vi "cdaq_test.vi"() -> ()   [LabVIEW 2013]
uses:
  cdaq_anal_session.ctl
  cdaq_anal_adc_command.ctl
  cdaq_anal_adc_data.ctl
panel:
  out "error out 2":errorcluster
  out "timestamp [s]":dbl
  out "adc data":dbl[](graph)
  in  "ADC N":i32
  in  "btn adc get":bool
  in  "btn set dac":bool
  in  "amp":sgl
  in  "ws":sgl
  in  "N":i32
  in  "btn stop":bool
  out "error out":errorcluster
  in  "cdaq session in":T1={"mclk [Hz]"=12800000.0, "DAC device"="cDAQ2Mod7", "ADC device"="cDAQ2Mod8", "DAC task"="", "ADC task"="", "adc idn"="", "dac idn"="", "fs [Hz]"=50000.0, "queue adc cmd"=refnum, "queue adc data"=refnum, "adc proc ref"=refnum}
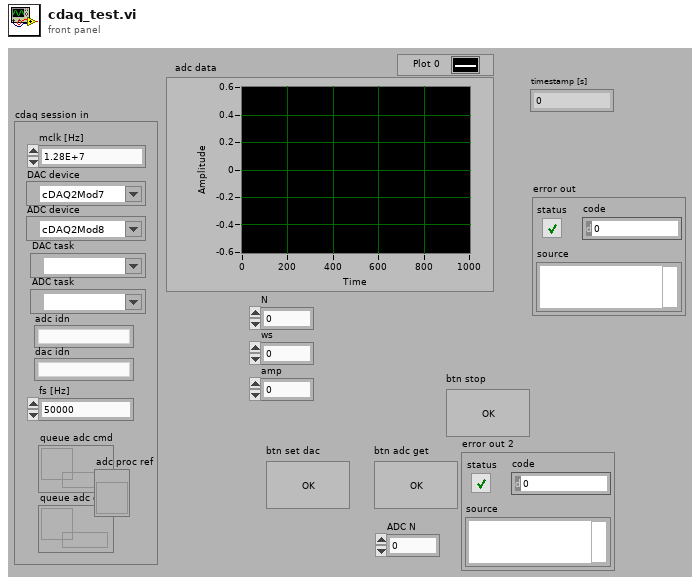
[diagram p1: front panel]
types:
  T1 = typedef "cdaq_anal_session.ctl" = cluster{"mclk [Hz]":dbl, "DAC device":tag, "ADC device":tag, "DAC task":refnum<k21>, "ADC task":refnum<k21>, "adc idn":string, "dac idn":string, "fs [Hz]":dbl, "queue adc cmd":refnum<queue>, "queue adc data":refnum<queue>, "adc proc ref":refnum<vi>}
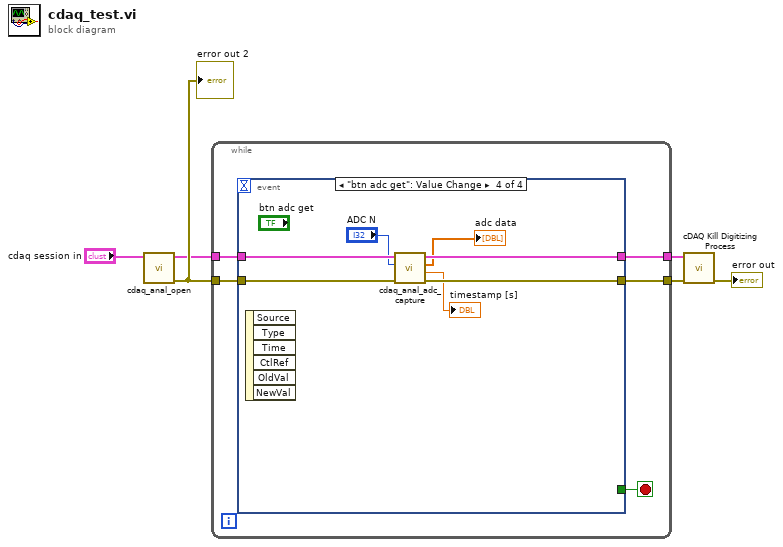
[diagram p0: block diagram]
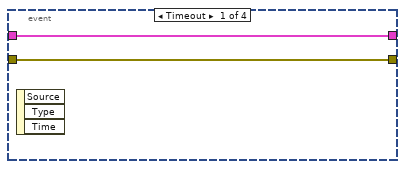
[diagram p2: hidden frame]
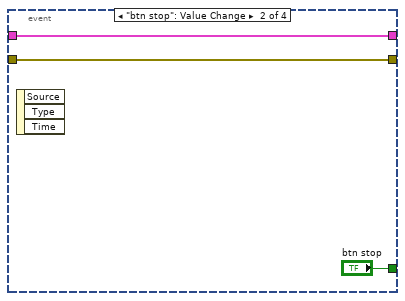
[diagram p3: hidden frame]
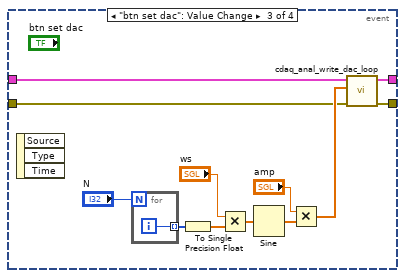
[diagram p4: hidden frame]
diagram:
  n1 = call "cdaq_anal_open.vi"("cdaq session in"="cdaq session in") -> ("error out"=w3:errorcluster, "cdaq session out"=w2:T1)  [unwired: 7 in, 2 out]
  "error out 2" <- w3
  n2 = while {
    tunnel: [w11] -> w5
    tunnel: w3 -> [w10]
    tunnel: w2 -> [w9]
    tunnel: [w8] -> w1
    stop <- w7 stop-if-true
    n3 = event shown="[3] \"btn adc get\": Value Change" {
      selector: _ -> [_ _ _ _]
      dyn-events: _ -> [_ _ _ _]
      timeout: _ -> [_ _ _ _]
      tunnel: [w13 w15 w20 w34] -> w11
      tunnel: w10 -> [w13 w15 w19 w36]
      tunnel: w9 -> [w12 w16 w18 w35]
      tunnel: [w12 w16 w17 w33] -> w8
      tunnel: [_ "btn stop" _ _] -> w7
      event Timeout {
        n4 = event-data() -> ()  [unwired: 1 in, 3 out]
      }
      event "btn stop": Value Change {
        n5 = event-data() -> ()  [unwired: 1 in, 3 out]
      }
      event "btn set dac": Value Change {
        n6 = event-data() -> ()  [unwired: 1 in, 3 out]
        n7 = for {
          N: "N" -> [_]
          tunnel: [w29] -> w22 mode=indexing
          i -> [w29]
        }
        n8 = To Single Precision Float(number=w22) -> (single precision float=w23:sgl[])
        n9 = Multiply(x="ws", y=w23) -> (x*y=w25:sgl[])
        n10 = Sine(x=w25) -> (sin(x)=w26:sgl[])
        n11 = Multiply(x="amp", y=w26) -> (x*y=w28:sgl[])
        n12 = call "cdaq_anal_write_dac_loop.vi"("error in"=w19, "wave"=w28, "cdaq session in"=w18) -> ("error out"=w20:errorcluster, "cdaq session out"=w17:T1)  [unwired: 6 in, 1 out]
      }
      event "btn adc get": Value Change {
        n13 = event-data() -> ()  [unwired: 1 in, 6 out]
        n14 = call "cdaq_anal_adc_capture.vi"("error in"=w36, "N"="ADC N", "cdaq session in"=w35) -> ("error out"=w34:errorcluster, "timestamp [s]"=→"timestamp [s]":dbl, "wave"=→"adc data":dbl[], "cdaq session out"=w33:T1)  [unwired: 5 in]
      }
    }
  }
  n15 = call "cDAQ Kill Digitizing Process.vi"("error in"=w5, "cdaq session in"=w1) -> ("error out"=→"error out":errorcluster)  [unwired: 8 in, 1 out]
